vi "Log State.vi"(8 "error in (no error)":errorcluster, 10 "Model Status":T3, 11 "Data":T1) -> (0 "error out":errorcluster, 3 "Data out":T1)   [LabVIEW 2015, in "Logger.lvlib"]
uses:
  Logger.lvlib
  PL Model/API/Get Model Status Control.ctl
  TypeDefs/Logger Data.ctl
  TypeDefs/Logger State.ctl
  PL Model/PL Model.lvlib
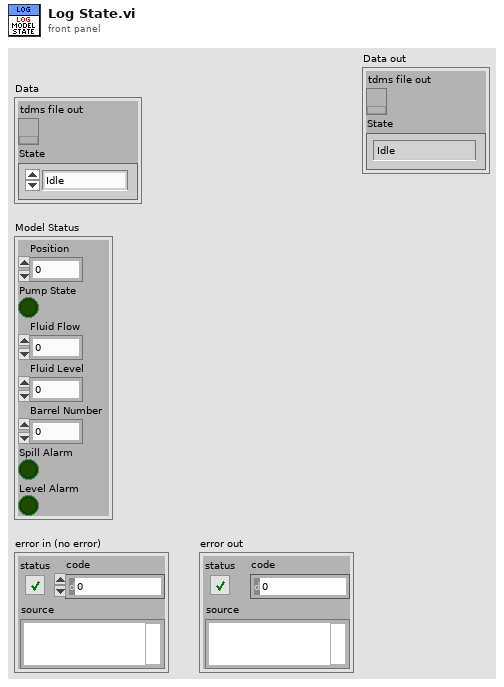
[diagram p1: front panel]
types:
  T1 = typedef "Logger.lvlib/Logger Data.ctl" = cluster{"tdms file out":refnum<k34>, "State":T2}
  T2 = typedef "Logger.lvlib/Logger State.ctl" = enum16{"Idle", "Working"}
  T3 = typedef "PL Model.lvlib/Get Model Status Control.ctl" = cluster{"Position":dbl, "Pump State":bool, "Fluid Flow":dbl, "Fluid Level":dbl, "Barrel Number":i32, "Spill Alarm":bool, "Level Alarm":bool}
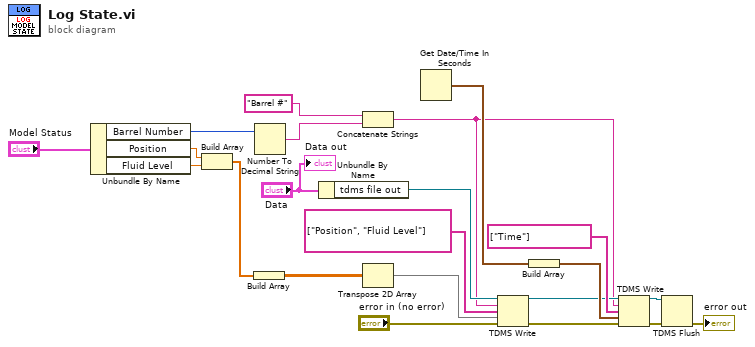
[diagram p0: block diagram]
diagram:
  n1 = Unbundle By Name("Model Status") -> ("Barrel Number"=w4:i32, "Position"=w10:dbl, "Fluid Level"=w11:dbl)
  n2 = Build Array(w10, w11) -> (w17:dbl[])
  n3 = Build Array(w17) -> (w18:dbl[][])
  n4 = Number To Decimal String(number=w4) -> (decimal integer string=w2:string)  [unwired: 1 in]
  n5 = Unbundle By Name("Data") -> ("tdms file out"=w8:refnum<k34>)
  n6 = Concatenate Strings("Barrel #", w2) -> (w1:string)
  n7 = Transpose 2D Array(2D array=w18) -> (transposed array=w19:dbl[][])
  n8 = Get Date/Time In Seconds() -> (seconds since 1Jan1904=w15:timestamp)
  n9 = TDMS Write(0:w8, 5:w1, 7:string[] ["Position", "Fluid Level"], 9:w19, 11:"error in (no error)") -> (4:w13:refnum<k34>, 15:w12:errorcluster)  [unwired: 1 in, 2 out]
  n10 = Build Array(w15) -> (w16:timestamp[])
  n11 = TDMS Write(0:w13, 5:w1, 7:string[] ["Time"], 9:w16, 11:w12) -> (4:w21:refnum<k34>, 15:w20:errorcluster)  [unwired: 1 in, 2 out]
  n12 = TDMS Flush(4:w20, 7:w21) -> (0:→"error out":errorcluster)  [unwired: 1 out]
  "Data out" <- "Data"
